vi "SaveMCSAFFTData.vi"(6 "Registry":T16, 7 "data event data":T1, 8 "error in (no error)":errorcluster, 10 "MCSA FFT":T9, 11 "data event":T10) -> (0 "error out":errorcluster, 3 "data event data out":T1)   [LabVIEW 2017, in "McsaDataEventCreator.lvlib"]
uses:
  <vilib>/addons/InsightCM/Devices/Shared/Mcsa/McsaDataEventCreator/McsaDataEventCreator.lvlib
  <vilib>/addons/InsightCM/Devices/Shared/Mcsa/McsaDataEventCreator/controls/DataGroupRegistry.ctl
  <vilib>/addons/InsightCM/Devices/Shared/Mcsa/McsaDataEventCreator/controls/Registry_DataSet.ctl
  <vilib>/addons/InsightCM/Devices/Shared/Mcsa/McsaDataEventCreator/controls/DataSetType.ctl
  <vilib>/addons/InsightCM/Devices/Shared/Common/DataEventCreator/controls/Registry_Trend.ctl
  <vilib>/addons/InsightCM/Devices/Shared/Mcsa/McsaDataEventCreator/controls/DataEventConfig.ctl
  <vilib>/addons/InsightCM/Devices/Shared/Mcsa/McsaDataEventCreator/controls/AcqParams.ctl
  <vilib>/addons/InsightCM/Devices/Shared/Common/DataAccumulator/controls/AccumulationSettings.ctl
  <vilib>/addons/InsightCM/Devices/Shared/Common/DataAccumulator/controls/accumulationType.ctl
  <vilib>/addons/InsightCM/Devices/Shared/Common/DVRBuffer/controls/BufferLocation.ctl
  <vilib>/addons/PointValueMap/controls/PointMap.ctl
  <vilib>/addons/InsightCM/Utilities/Analysis/MCSA/controls/McsaFFT.ctl
  <vilib>/addons/InsightCM/Devices/Shared/Common/DataEvent/controls/Event.ctl
  <vilib>/addons/InsightCM/MessageBus/Base/controls/DataEvent.ctl
  <vilib>/addons/InsightCM/MessageBus/Base/controls/KeyValuePair.ctl
  <vilib>/addons/InsightCM/Devices/Shared/Common/DataEvent/controls/DataSet.ctl
  <vilib>/addons/InsightCM/MessageBus/Base/controls/DataSetMetadata.ctl
  <vilib>/addons/InsightCM/MessageBus/Base/controls/TrendPoint.ctl
  <vilib>/addons/InsightCM/MessageBus/Base/controls/TrendAlarmUpdate.ctl
  <vilib>/addons/InsightCM/MessageBus/Base/controls/TrendAlarmTransition.ctl
  <vilib>/addons/InsightCM/Utilities/MCSA/McsaUtilities.lvlib
  <vilib>/addons/PointValueMap/PointValueMap.lvlib
  <vilib>/addons/InsightCM/Devices/Shared/Common/DataEventCreator/DataEventCreator.lvlib
  <vilib>/addons/InsightCM/Devices/Shared/Common/DataAccumulator/DataAccumulator.lvlib
  <vilib>/addons/InsightCM/Devices/Shared/Common/DVRBuffer/DVRBuffer.lvlib
  <vilib>/addons/InsightCM/Utilities/Analysis/MCSA/McsaAnalysisFunctions.lvlib
  <vilib>/addons/InsightCM/Devices/Shared/Common/DataEvent/DataEvent.lvlib
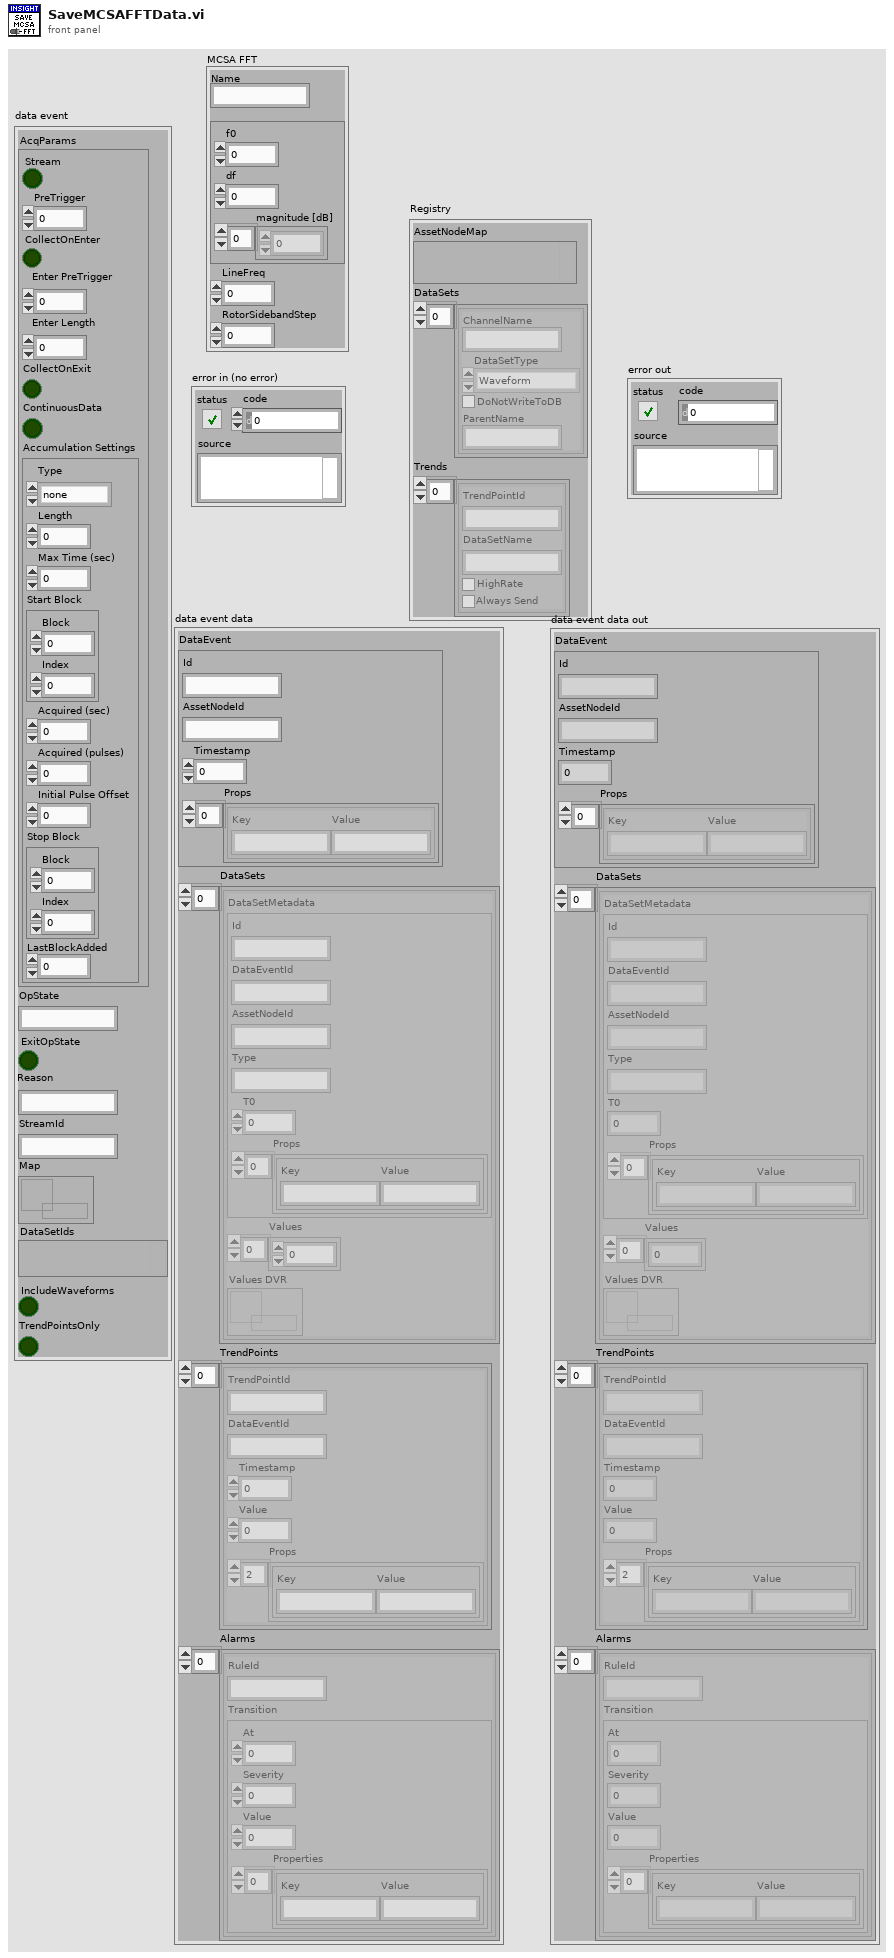
[diagram p1: front panel]
types:
  T1 = typedef "DataEvent.lvlib/Event.ctl" = cluster{"DataEvent":T2, "DataSets":T4[], "TrendPoints":T6[], "Alarms":T7[]}
  T2 = typedef "DataEvent.ctl" = cluster{"Id":string, "AssetNodeId":string, "Timestamp":i64, "Props":T3[]}
  T3 = typedef "KeyValuePair.ctl" = cluster{"Key":string, "Value":string}
  T4 = typedef "DataEvent.lvlib/DataSet.ctl" = cluster{"DataSetMetadata":T5, "Values":sgl[], "Values DVR":refnum<data-value>}
  T5 = typedef "DataSetMetadata.ctl" = cluster{"Id":string, "DataEventId":string, "AssetNodeId":string, "Type":string, "T0":i64, "Props":T3[]}
  T6 = typedef "TrendPoint.ctl" = cluster{"TrendPointId":string, "DataEventId":string, "Timestamp":i64, "Value":dbl, "Props":T3[]}
  T7 = typedef "TrendAlarmUpdate.ctl" = cluster{"RuleId":string, "Transition":T8}
  T8 = typedef "TrendAlarmTransition.ctl" = cluster{"At":i64, "Severity":i32, "Value":dbl, "Properties":T3[]}
  T9 = typedef "McsaAnalysisFunctions.lvlib/McsaFFT.ctl" = cluster{"Name":string, "Spectrum":cluster{"f0":dbl, "df":dbl, "magnitude [dB]":dbl[]}, "LineFreq":dbl, "RotorSidebandStep":dbl}
  T10 = typedef "McsaDataEventCreator.lvlib/DataEventConfig.ctl" = cluster{"AcqParams":T11, "OpState":string, "ExitOpState":bool, "Reason":string, "StreamId":string, "Map":T15, "DataSetIds":variant, "IncludeWaveforms":bool, "TrendPointsOnly":bool}
  T11 = typedef "McsaDataEventCreator.lvlib/AcqParams.ctl" = cluster{"Stream":bool, "PreTrigger":i32, "CollectOnEnter":bool, "Enter PreTrigger":i32, "Enter Length":dbl, "CollectOnExit":bool, "ContinuousData":bool, "Accumulation Settings":T12}
  T12 = typedef "DataAccumulator.lvlib/AccumulationSettings.ctl" = cluster{"Type":T13, "Length":dbl, "Max Time (sec)":dbl, "Start Block":T14, "Acquired (sec)":dbl, "Acquired (pulses)":i32, "Initial Pulse Offset":dbl, "Stop Block":T14, "LastBlockAdded":u32}
  T13 = typedef "DataAccumulator.lvlib/accumulationType.ctl" = enum16{"none", "seconds", "revolutions"}
  T14 = typedef "DVRBuffer.lvlib/BufferLocation.ctl" = cluster{"Block":u32, "Index":i32}
  T15 = typedef "PointValueMap.lvlib/PointMap.ctl" = refnum<data-value>
  T16 = typedef "McsaDataEventCreator.lvlib/DataGroupRegistry.ctl" = cluster{"AssetNodeMap":variant, "DataSets":T17[], "Trends":T19[]}
  T17 = typedef "McsaDataEventCreator.lvlib/Registry_DataSet.ctl" = cluster{"ChannelName":string, "DataSetType":T18, "DoNotWriteToDB":bool, "ParentName":string}
  T18 = typedef "McsaDataEventCreator.lvlib/DataSetType.ctl" = enum16{"Waveform", "MCSAFFT", "TorqueWFM"}
  T19 = typedef "DataEventCreator.lvlib/Registry_Trend.ctl" = cluster{"TrendPointId":string, "DataSetName":string, "HighRate":bool, "Always Send":bool}
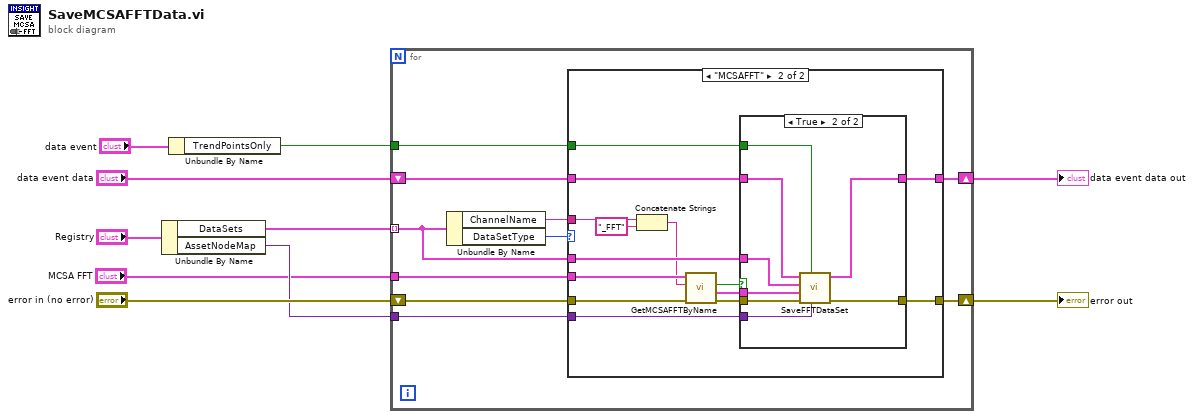
[diagram p0: block diagram]
diagram:
  n1 = Unbundle By Name("Registry") -> ("DataSets"=w8:T17[], "AssetNodeMap"=w6:variant)
  n2 = Unbundle By Name("data event") -> ("TrendPointsOnly"=w5:bool)
  n3 = for {
    tunnel: "MCSA FFT" -> [w19]
    tunnel: w8 -> [w13] mode=indexing
    shift-right: [w18] -> w7
    shift-left: "error in (no error)" -> [w20]
    tunnel: w6 -> [w14]
    shift-right: [w12] -> w1
    shift-left: "data event data" -> [w15]
    tunnel: w5 -> [w11]
    n4 = Unbundle By Name(w13) -> ("ChannelName"=w17:string, "DataSetType"=w16:T18)
    n5 = case shown="\"MCSAFFT\"" w16 {
      tunnel: w20 -> [w21 w31]
      tunnel: w19 -> [_ w29]
      tunnel: [w21 w36] -> w18
      tunnel: w17 -> [_ w25]
      tunnel: w15 -> [w22 w35]
      tunnel: w14 -> [_ w34]
      tunnel: w13 -> [_ w33]
      tunnel: [w22 w32] -> w12
      tunnel: w11 -> [_ w27]
      frame Default {
      }
      frame "MCSAFFT" {
        n6 = Concatenate Strings(w25, "_FFT" ("string")) -> (w24:string)
        n7 = call <vilib>:"GetMCSAFFTByName.vi"("error in (no error)"=w31, "Channel Name"=w24, "MCSA FFT in"=w29) -> ("error out"=w30:errorcluster, "MCSA FFT out"=w28:T9, "Found?"=w26:bool)  [unwired: 6 in]
        n8 = case shown="True" w26 {
          tunnel: w30 -> [w38 w46]
          tunnel: w28 -> [_ w45]
          tunnel: [w38 w40] -> w36
          tunnel: w35 -> [w37 w44]
          tunnel: w34 -> [_ w43]
          tunnel: w33 -> [_ w42]
          tunnel: [w37 w41] -> w32
          tunnel: w27 -> [_ w39]
          frame False {
          }
          frame True {
            n9 = call <vilib>:"SaveFFTDataSet.vi"("AssetNodeMap"=w43, "do not write to database"=w39, "error in (no error)"=w46, "MCSA FFT"=w45, "DataSetRegistry"=w42, "event in"=w44) -> ("error out"=w40:errorcluster, "event out"=w41:T1)  [unwired: 4 in]
          }
        }
      }
    }
  }
  "error out" <- w7
  "data event data out" <- w1
